vi "Action.vi"(8 "error in (no error)":errorcluster, 10 "Action":string, 11 "HarnessInterface in":refnum<class "lv_icon_class.lvclass">) -> (0 "error out":errorcluster, 3 "HarnessInterface out":refnum<class "lv_icon_class.lvclass">)   [LabVIEW 2021, in "lv_icon_class.lvclass"]
uses:
  <vilib>/LabVIEW Icon API/lv_icon/lv_icon_class/lv_icon_class.lvclass
  <vilib>/LabVIEW Icon API/lv_icon/lv_icon_class/lv_icon_class.lvclass/lv_icon_class.ctl
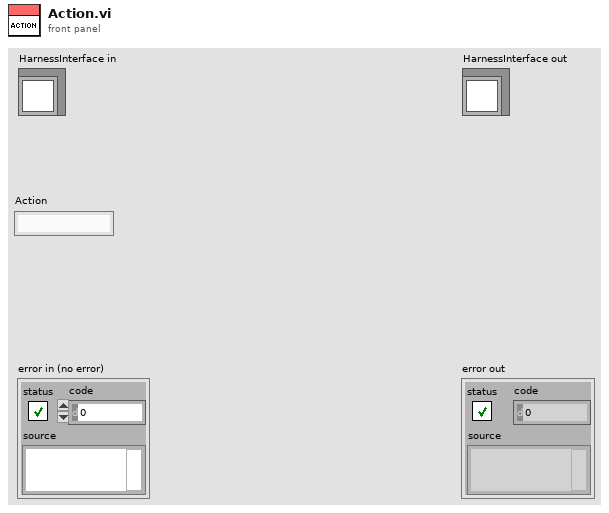
[diagram p1: front panel]
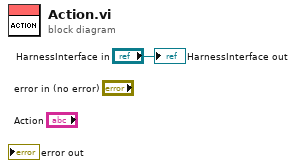
[diagram p0: block diagram]
diagram:
  "HarnessInterface out" <- "HarnessInterface in"
